vi "Stop Core.vi"(10 "final error code":i32, 11 "Samples in":refnum<class "Samples.lvclass">) -> (3 "Samples out":refnum<class "Samples.lvclass">)   [LabVIEW 2015, in "AMS UI.lvlib" / "Samples.lvclass"]
doc: "(<B>Filename</B>: Actor Framework.lvlib:Actor.lvclass:Stop Core.vi)\n\nDefines what the actor does before it stops. Use the <B>final error code</B> input to determine whether the actor shut down in response to an error.\n\nBy default, this method does nothing. A descendant class may override it to define behavior, such as shutting down any processes the actor initiated in its override of the Actor Core method."
uses:
  Samples.lvclass
  Samples.lvclass/Samples.ctl
  AMS Gas Actor/AMS Gas Actor.lvclass
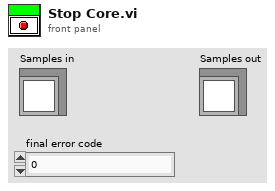
[diagram p1: front panel]
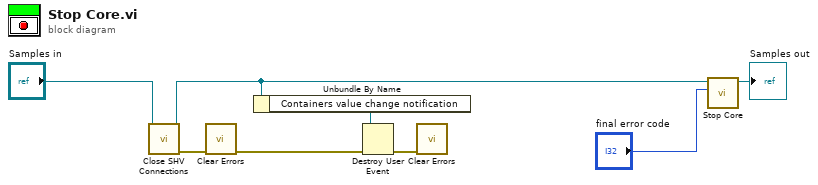
[diagram p0: block diagram]
diagram:
  n1 = call "Close SHV Connections.vi"("Samples in"="Samples in") -> ("error out"=w5:errorcluster, "Samples out"=w4:refnum<class "Samples.lvclass">)  [unwired: 9 in]
  n2 = call <vilib>:"Clear Errors.vi"("error in (no error)"=w5) -> ("error out"=w2:errorcluster)  [unwired: 5 in, 1 out]
  n3 = Unbundle By Name(w4) -> ("Containers value change notification"=w3:refnum<user-event>)
  n4 = Destroy User Event(user event=w3, error in=w2) -> (error out=w1:errorcluster)
  n5 = call <vilib>:"Clear Errors.vi"("error in (no error)"=w1) -> ()  [unwired: 5 in, 2 out]
  n6 = call-parent "Stop Core.vi"("final error code"="final error code", "AMS Gas Actor in"=w4) -> ("AMS Gas Actor out"=→"Samples out":refnum<class "Samples.lvclass">)  [unwired: 9 in]
